vi "APS get sampling param ex.vi"(8 "error in (no error)":errorcluster caption="错误输入（无错误）", 10 "Param":T1, 11 "Board_ID":i32) -> (0 "error out":errorcluster caption="错误输出", 2 "Param out":T1, 3 "function return":i32)   [LabVIEW 2011, in "APS168.lvlib"]
doc: "I32 FNTYPE APS_get_sampling_param_ex( I32 Board_ID, SAMP_PARAM *Param );"
uses:
  APS168.lvlib
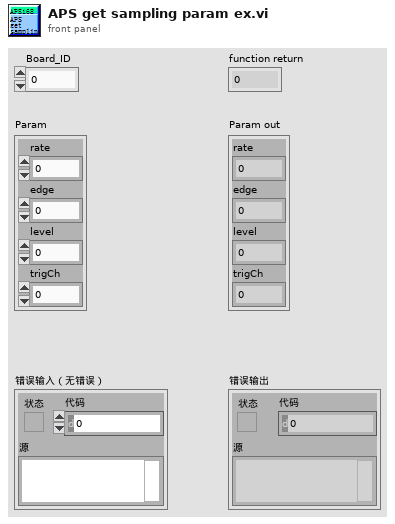
[diagram p1: front panel]
types:
  T1 = cluster{"rate":i32, "edge":i32, "level":i32, "trigCh":i32}
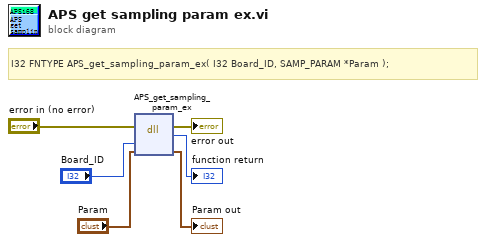
[diagram p0: block diagram]
diagram:
  # "I32 FNTYPE APS_get_sampling_param_ex( I32 Board_ID, SAMP_PARAM *Param );"
  n1 = dll-call lib="PTH1Labs E软件ADLINK 204CAPS_1_7_1_LIB line 连续运动204APS168.*" fn="APS_get_sampling_param_ex"(error in="error in (no error)", "Board_ID"="Board_ID", "Param"="Param") -> (error out=→"error out":errorcluster, →"function return":i32, "Param"=→"Param out":T1)  [unwired: 3 in, 1 out]
